vi "Dail Strip Dn_Barcode read.vi"(8 "error in":errorcluster, 11 "queue in":refnum<queue>) -> (0 "error out":errorcluster, 1 "exit":bool, 2 "read buffer":string, 3 "queue Out 2":refnum<queue>)   [LabVIEW 2015]
uses:
  Test  enqueue/AutoTest seq.ctl
  <vilib>/Instr/_visa.llb/VISA Configure Serial Port (Instr).vi
  Galobal variable_TI.vi
  Project Setup/Globle Variable/GR_Servo.vi
panel:
  out "x = y?":bool
  out "substring":string
  out "error out 2":errorcluster
  out "error out":errorcluster
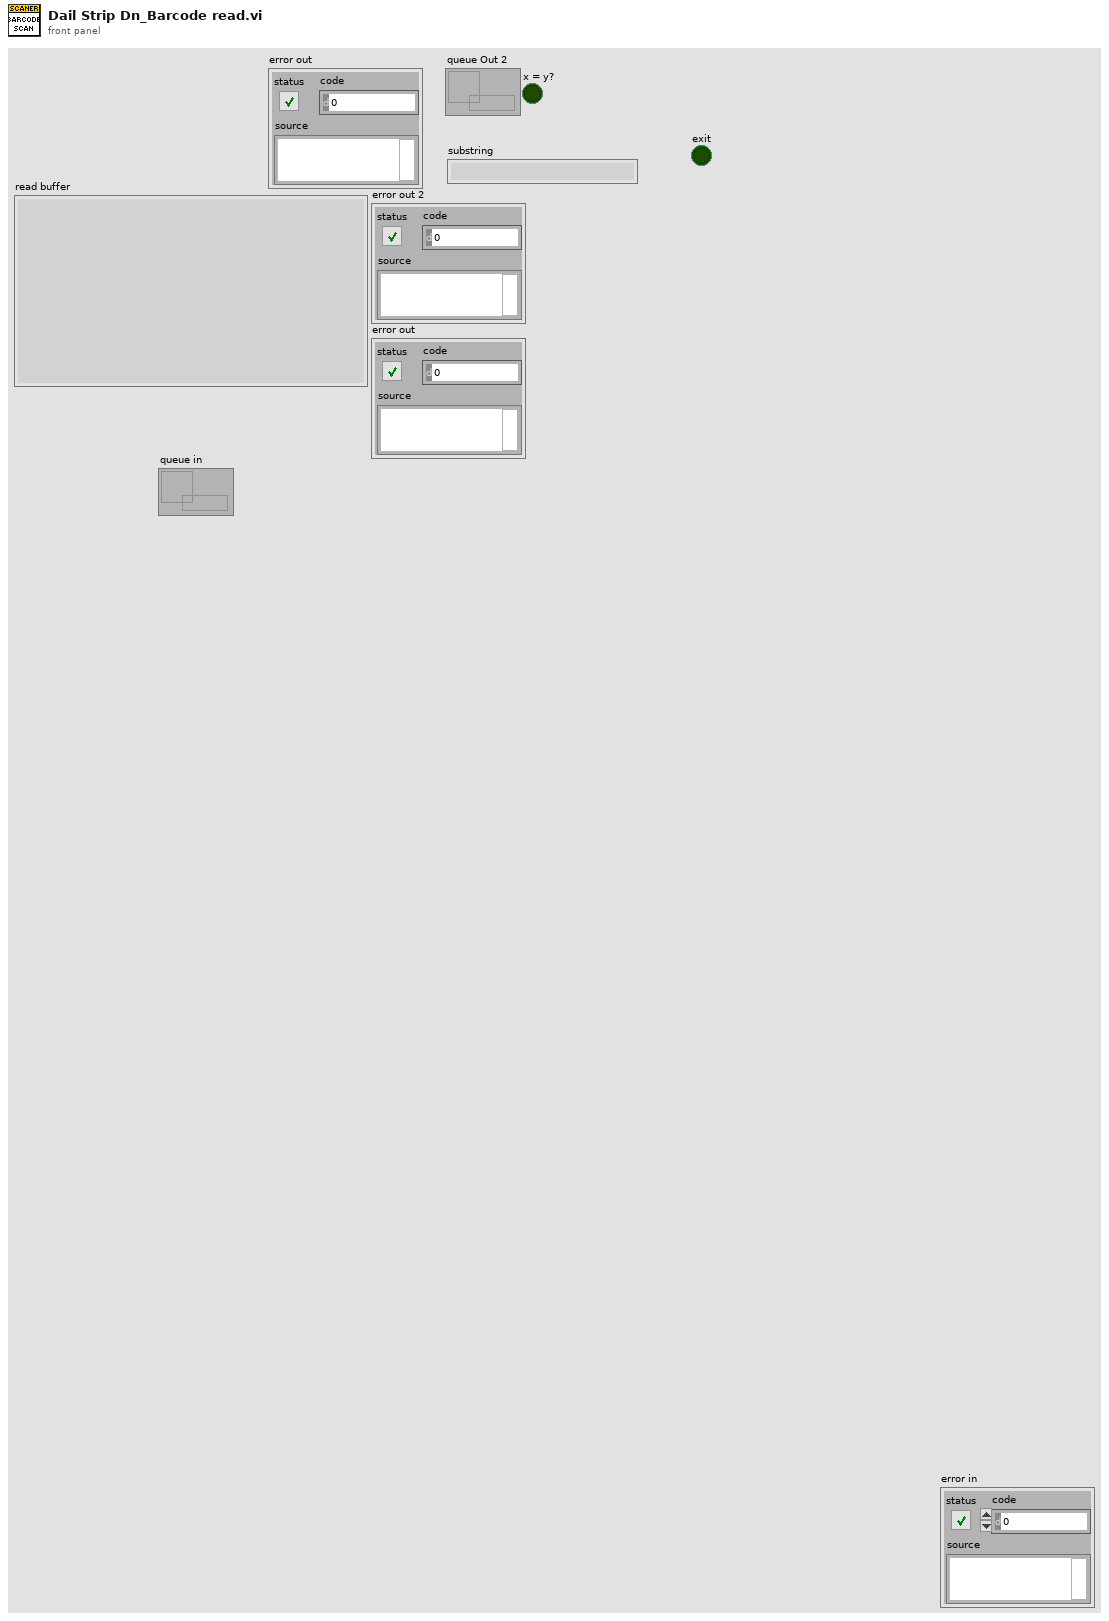
[diagram p1: front panel]
types:
  T1 = cluster{"MaxLoad(N) ":dbl, "Min Load(N)":dbl, "Load Offset":dbl, "Model":string, "MIC Code":string, "Dial Speedo":string, "Dial RMP":string, "Blinker":string, "Telltale":string}
  T2 = cluster{"Start":bool, "Emergency ":bool, "Reset":bool, "Home":bool, "Safety":bool}
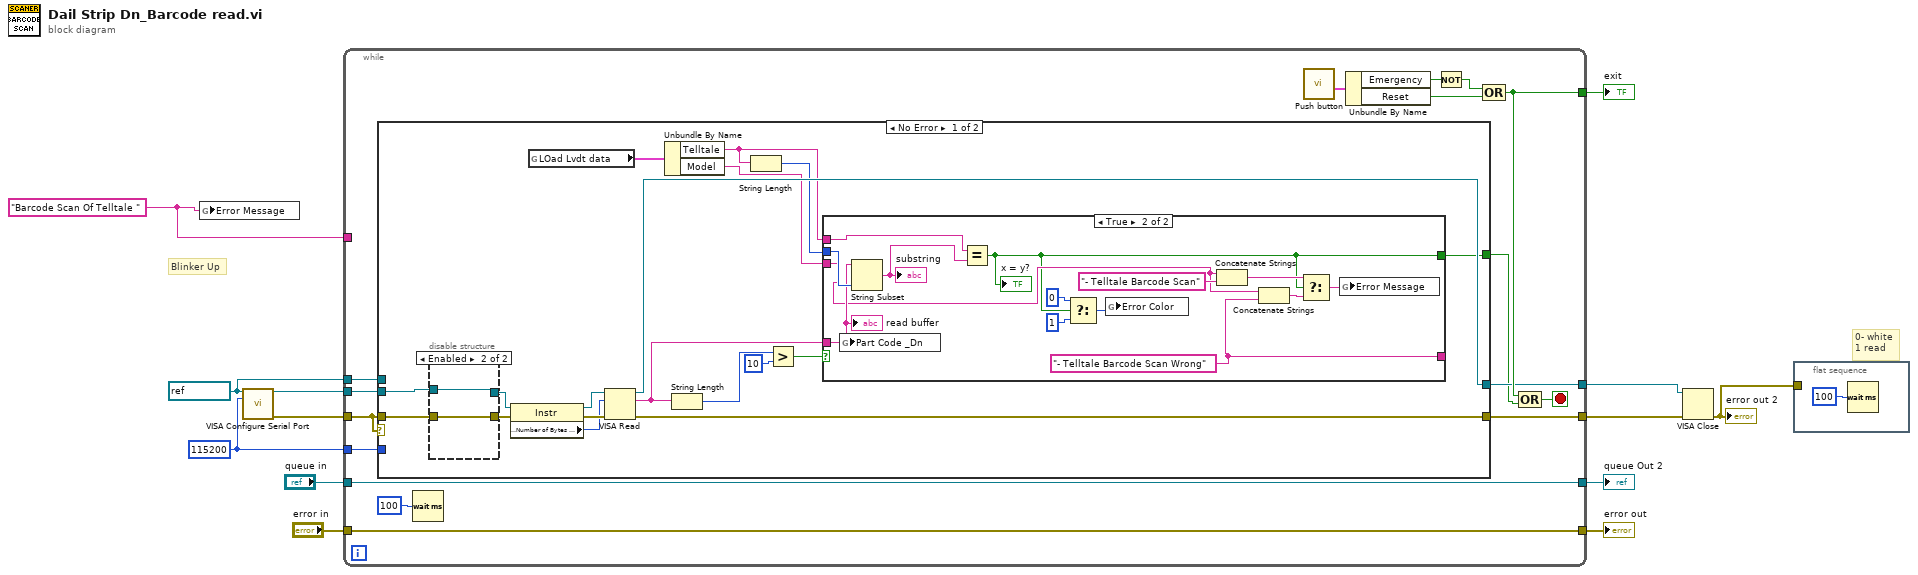
[diagram p0: block diagram]
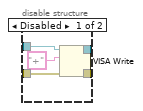
[diagram p2: hidden frame]
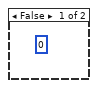
[diagram p3: hidden frame]
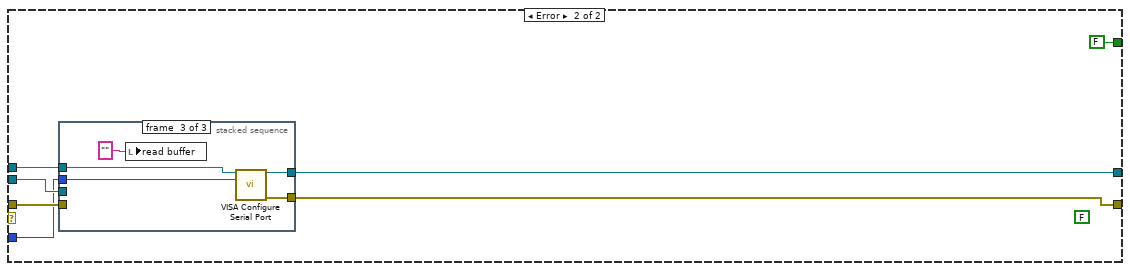
[diagram p4: hidden frame]
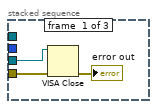
[diagram p5: hidden frame]
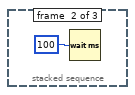
[diagram p6: hidden frame]
diagram:
  w1 = "Barcode Scan Of Telltale " ("string")
  w8 = u32 115200 ("baud rate (9600)")
  w9 = refnum<visa-resource-name> "COM2" ("VISA resource name")
  # "Blinker Up"
  # "0- white\n1 read"
  n1 = global write "GR_Servo.vi" "Error Message"(w1) -> ()
  n2 = call-poly "VISA Configure Serial Port"("VISA resource name"=w9, "baud rate (9600)"=w8) -> ("VISA resource name out"=w13:refnum<visa-resource-name>, "error out"=w12:errorcluster)  [unwired: 12 in]
  n3 = while {
    tunnel: w13 -> [w29]
    tunnel: w12 -> [w27]
    tunnel: [w15] -> w11
    tunnel: [w28] -> w10
    tunnel: w9 -> [w26]
    tunnel: w8 -> [w25]
    tunnel: [w16] -> w7
    tunnel: [w22] -> w5
    tunnel: "queue in" -> [w22]
    tunnel: "error in" -> [w21]
    tunnel: [w21] -> w3
    tunnel: w1 -> [_]
    stop <- w23 stop-if-true
    n4 = case shown="No Error" w27 {
      tunnel: w29 -> [w47 w75]
      tunnel: w27 -> [w46 w74]
      tunnel: [w45 w71] -> w15
      tunnel: [w44 w70] -> w28
      tunnel: w26 -> [_ w73]
      tunnel: w25 -> [_ w72]
      tunnel: [w30 FALSE] -> w14
      frame No Error {
        n5 = disable-structure shown="Enabled" {
          disable-tunnel: w47 -> [w52 w54]
          disable-tunnel: w46 -> [w51 w53]
          disable-tunnel: [w50 w53] -> w43
          disable-tunnel: [w49 w54] -> w42
          frame Disabled {
            n6 = VISA Write(VISA resource name=w52, write buffer="+", error in (no error)=w51) -> (VISA resource name out=w49:refnum<visa-resource-name>, error out=w50:errorcluster)  [unwired: 1 out]
          }
          frame Enabled {
          }
        }
        n7 = property class="Instr"(reference=w42, error in=w43) -> (reference out=w41:refnum<visa-resource-name>, error out=w40:errorcluster, "Serial Settings:Number of Bytes at Serial Port"=w39:u32)
        n8 = global read "Galobal variable_TI.vi" "LOad Lvdt data"() -> (w34:T1)
        n9 = VISA Read(VISA resource name=w41, byte count=w39, error in (no error)=w40) -> (VISA resource name out=w45:refnum<visa-resource-name>, read buffer=w36:string, error out=w44:errorcluster)  [unwired: 1 out]
        n10 = Unbundle By Name(w34) -> ("Telltale"=w33:string, "Model"=w31:string)
        n11 = String Length(string=w36) -> (length=w38:i32)
        n12 = String Length(string=w33) -> (length=w32:i32)
        n13 = Greater?(x=w38, y=10) -> (0:w35:bool)
        n14 = case shown="True" w35 {
          tunnel: w36 -> [_ w63]
          tunnel: w33 -> [_ w67]
          tunnel: w32 -> [_ w68]
          tunnel: w31 -> [_ w56]
          tunnel: [_ w55] -> w30
          tunnel: [_ w57] -> _
          frame False {
            (unwired) 0 ("f")
          }
          frame True {
            w57 = "- Telltale Barcode Scan Wrong" ("string")
            n15 = global write "Galobal variable_TI.vi" "Part Code _Dn"(w63) -> ()
            n16 = String Subset(string=w63, length (rest)=w68) -> (substring=w66:string)  [unwired: 1 in]
            "substring" <- w66
            n17 = Equal?(x=w67, y=w66) -> (x = y?=w55:bool)
            "x = y?" <- w55
            n18 = Select(t=0, s=w55, f=1) -> (s? t:f=w62:i32)
            n19 = global write "GR_Servo.vi" "Error Color"(w62) -> ()
            n20 = Concatenate Strings(w56, "- Telltale Barcode Scan" ("string")) -> (w60:string)
            n21 = Concatenate Strings(w56, w57) -> (w59:string)
            n22 = Select(t=w60, s=w55, f=w59) -> (s? t:f=w58:string)
            n23 = global write "GR_Servo.vi" "Error Message"(w58) -> ()
            "read buffer" <- w63
          }
        }
      }
      frame Error {
        (unwired) FALSE
        n24 = stacked-sequence {
          tunnel: w75 -> [w77 _ _]
          tunnel: w74 -> [w76 _ _]
          tunnel: w73 -> [_ _ w84]
          tunnel: w72 -> [_ _ w83]
          tunnel: [_ _ w82] -> w71
          tunnel: [_ _ w81] -> w70
          frame #0 {
            n25 = VISA Close(VISA resource name=w77, error in (no error)=w76) -> (error out=→"error out":errorcluster)
          }
          frame #1 {
            n26 = Wait (ms)(milliseconds to wait=u32 100) -> ()  [unwired: 1 out]
          }
          frame #2 {
            n27 = local write "read buffer"("" ("read buffer")) -> ()
            n28 = call-poly "VISA Configure Serial Port"("VISA resource name"=w84, "baud rate (9600)"=w83) -> ("VISA resource name out"=w82:refnum<visa-resource-name>, "error out"=w81:errorcluster)  [unwired: 12 in]
          }
        }
      }
    }
    n29 = Wait (ms)(milliseconds to wait=u32 100) -> ()  [unwired: 1 out]
    n30 = call "Push button.vi"() -> ("Push Button"=w20:T2)  [unwired: 9 in, 2 out]
    n31 = Unbundle By Name(w20) -> ("Emergency"=w19:bool, "Reset"=w17:bool)
    n32 = Not(x=w19) -> (.not. x?=w18:bool)
    n33 = Compound Arithmetic op=OR(w18, w17) -> (w16:bool)
    n34 = Compound Arithmetic op=OR(w16, w14) -> (w23:bool)
  }
  "exit" <- w7
  "queue Out 2" <- w5
  "error out" <- w3
  n35 = VISA Close(VISA resource name=w11, error in (no error)=w10) -> (error out=w2:errorcluster)
  "error out 2" <- w2
  n36 = flat-sequence {
    tunnel: w2 -> [_]
    frame #0 {
      n37 = Wait (ms)(milliseconds to wait=u32 100) -> ()  [unwired: 1 out]
    }
  }
